vi "checkChannelsCreated.vi"(8 "error in (no error)":errorcluster, 11 "Connection.TCP in":refnum<class "Connection.TCP.lvclass">) -> (0 "error out":errorcluster, 1 "outbound created":bool, 2 "inbound created":bool, 3 "Connection.TCP out":refnum<class "Connection.TCP.lvclass">)   [LabVIEW 2013, in "Connection.TCP_GOSPL.lvlib" / "Connection.TCP.lvclass"]
uses:
  Connection.TCP.lvclass
  Connection/Connection.lvclass
  Connection.TCP.lvclass/Connection.TCP.ctl
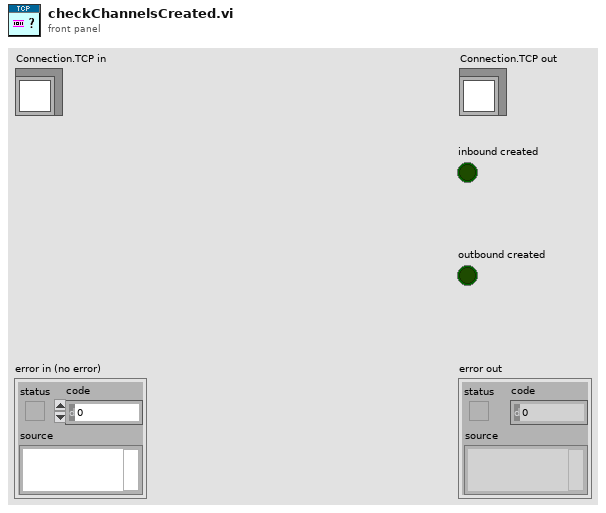
[diagram p1: front panel]
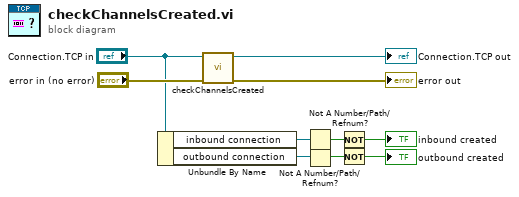
[diagram p0: block diagram]
diagram:
  n1 = Unbundle By Name("Connection.TCP in") -> ("inbound connection"=w7:refnum<k5>, "outbound connection"=w2:refnum<k5>)
  n2 = call-parent "checkChannelsCreated.vi"("error in (no error)"="error in (no error)", "Connection in"="Connection.TCP in") -> ("error out"=→"error out":errorcluster, "Connection out"=→"Connection.TCP out":refnum<class "Connection.TCP.lvclass">)  [unwired: 6 in, 2 out]
  n3 = Not A Number/Path/Refnum?(number/path/refnum=w7) -> (NaN/Path/Refnum?=w5:bool)
  n4 = Not A Number/Path/Refnum?(number/path/refnum=w2) -> (NaN/Path/Refnum?=w3:bool)
  n5 = Not(x=w5) -> (.not. x?=→"inbound created":bool)
  n6 = Not(x=w3) -> (.not. x?=→"outbound created":bool)
